vi "ReadHTTPHeader.vi"(8 "error in (no error)":errorcluster, 9 "timeout ms (25000)":i32=25000, 11 "WebSocket in":refnum<class "WebSocket.lvclass">) -> (0 "error out":errorcluster, 2 "HTTP Header":string, 3 "WebSocket out":refnum<class "WebSocket.lvclass">)   [LabVIEW 2021, in "WebSockets.lvlib" / "WebSocket.lvclass"]
doc: "Reads a HTTP header (ending in \\r\\n\\r\\n) from the Socket connection.\nWebSockets 2.0.1.40\nSam Sharp - MediaMongrels Ltd\nCopyright (c) 2019, MediaMongrels Ltd"
uses:
  WebSocket.lvclass
  WebSocket.lvclass/WebSocket.ctl
  Sockets/Socket/Socket.lvclass
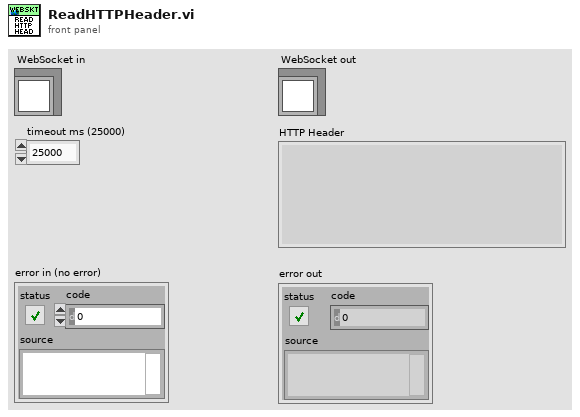
[diagram p1: front panel]
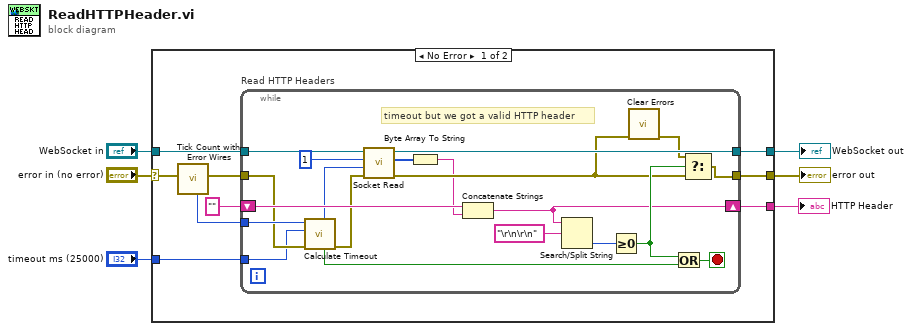
[diagram p0: block diagram]
diagram:
  n1 = case shown="No Error" "error in (no error)" {
    selector: "error in (no error)" -> [w7 w36]
    tunnel: [w14 w36] -> w6
    tunnel: "timeout ms (25000)" -> [w13 _]
    tunnel: "WebSocket in" -> [w12 w37]
    tunnel: [w11 w37] -> w3
    tunnel: [w10 _] -> w2
    frame No Error {
      n2 = call "Tick Count with Error Wires.vi"("error in (no error)"=w7) -> ("error out"=w9:errorcluster, "millisecond timer value"=w8:u32)  [unwired: 9 in]
      n3 = while "Read HTTP Headers" {
        tunnel: w12 -> [w35]
        tunnel: [w34] -> w11
        shift-right: [w24] -> w10
        shift-left: "" -> [w32]
        tunnel: w13 -> [w18]
        tunnel: [w25] -> w14
        tunnel: w9 -> [w19]
        tunnel: w8 -> [w20]
        stop <- w31 stop-if-true
        # "timeout but we got a valid HTTP header"
        n4 = call "Calculate Timeout.vi"("error in (no error)"=w19, "timeout ms"=w18, "t0"=w20) -> ("error out"=w21:errorcluster, "Elapsed?"=w17:bool, "new timeout ms"=w22:i32)  [unwired: 6 in]
        n5 = call "Socket Read.vi"("error in (no error)"=w21, "timeout ms (5000)"=w22, "# bytes to read"=1 ("bytes to read"), "WebSocket in"=w35) -> ("error out"=w23:errorcluster, "Read Bytes"=w33:u8[], "WebSocket out"=w34:refnum<class "WebSocket.lvclass">)  [unwired: 4 in, 1 out]
        n6 = Byte Array To String(unsigned byte array=w33) -> (string=w16:string)
        n7 = Concatenate Strings(w32, w16) -> (w24:string)
        n8 = Search/Split String(string=w24, search string/char (-)="\r\n\r\n") -> (offset of match=w30:i32)  [unwired: 1 in, 2 out]
        n9 = Greater Or Equal To 0?(x=w30) -> (x >= 0?=w27:bool)
        n10 = call <vilib>:"Clear Errors.vi"("error in (no error)"=w23) -> ("error out"=w26:errorcluster)  [unwired: 5 in, 1 out]
        n11 = Or(x=w27, y=w17) -> (x .or. y?=w31:bool)
        n12 = Select(t=w26, s=w27, f=w23) -> (s? t:f=w25:errorcluster)
      }
    }
    frame Error {
    }
  }
  "error out" <- w6
  "WebSocket out" <- w3
  "HTTP Header" <- w2
